vi "AWS_Core Set Credentials.vi"(8 "error in (no error)":errorcluster, 10 "AWS Credentials":T1, 11 "AWS_SQS in":refnum<class "AWS_SQS.lvclass">) -> (0 "error out":errorcluster, 3 "AWS_SQS out":refnum<class "AWS_SQS.lvclass">)   [LabVIEW 2012]
uses:
  AWS Core Lib/VI Source/Typedefs/AWS_AWS Credentials.ctl
  AWS Core Lib/VI Source/AWS_Core.lvlib
  AWS_SQS.lvclass
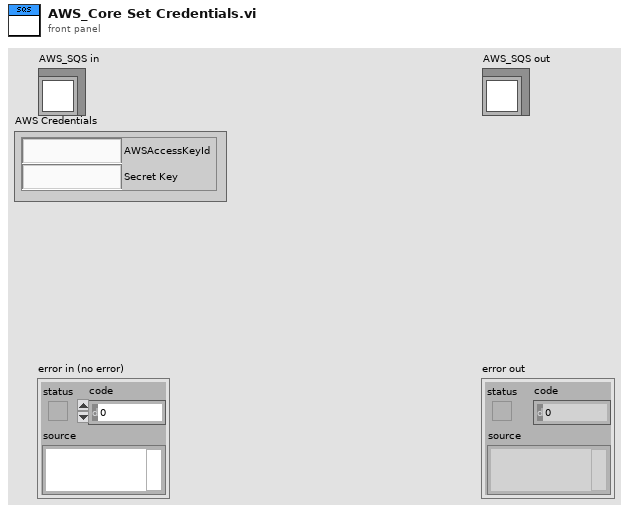
[diagram p1: front panel]
types:
  T1 = typedef "AWS_Core.lvlib/AWS_AWS Credentials.ctl" = cluster{"AWSAccessKeyId":string, "Secret Key":string}
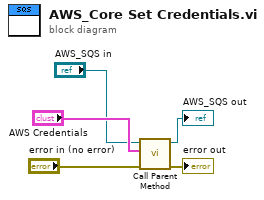
[diagram p0: block diagram]
diagram:
  n1 = call-parent "Call Parent Method"("error in (no error)"="error in (no error)", "AWS Credentials"="AWS Credentials", "AWS_Core in"="AWS_SQS in") -> ("error out"=→"error out":errorcluster, "AWS_Core out"=→"AWS_SQS out":refnum<class "AWS_SQS.lvclass">)  [unwired: 7 in]
